vi "Configure.vi"(8 "error in (no error)":errorcluster, 11 "MCCW ACLR in":refnum<class "MCCW ACLR.lvclass">) -> (0 "error out":errorcluster, 3 "MCCW ACLR out":refnum<class "MCCW ACLR.lvclass">)   [LabVIEW 2020, in "MCCW ACLR.lvclass"]
doc: "Configure the measurements paramaters to sweep.\nThis should be a pop up interface invoked by the configure test button on the main panel."
uses:
  MCCW ACLR.lvclass
  MCCW ACLR.lvclass/MCCW ACLR.ctl
  Controls/ACLR configuration.ctl
panel:
  in  "Signal BW [MHz]":dbl
  in  "Number of Carrieres":enum32{"From To", "Array"}(tab)
  in  "Carriers Cluster":cluster{"From":dbl, "To":dbl, "Step":dbl}
  in  "Carriers Array":dbl[](array[numeric]) format="%#_6p"
  in  "OK Button":bool
  in  "Number of Measurements":u32
  in  "MCCW Random Phase":bool
  in  "MCCW Phase Value":dbl min=0.0 max=360.0 step=0.01
  in  "Power":enum32{"From To", "Array"}(tab)
  in  "Power Cluster":cluster{"From":dbl, "To":dbl, "Step":dbl}
  in  "Power Array":dbl[](array[numeric]) format="%#_6p"
  in  "Frequency":enum32{"From To", "Array"}(tab)
  in  "Frequency Cluster":cluster{"From":dbl, "To":dbl, "Step":dbl}
  in  "Frequency Array":dbl[](array[numeric]) format="%#_6p"
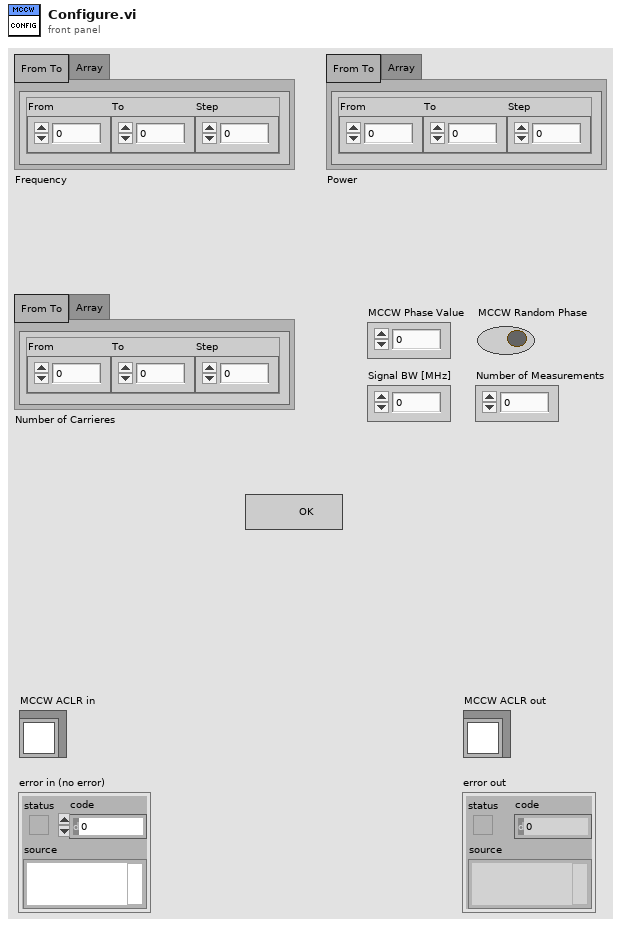
[diagram p1: front panel]
types:
  T1 = enum8{"Enabled", "Disabled", "Disabled and Grayed Out"}
  T2 = typedef "MCCW ACLR.lvclass/ACLR configuration.ctl" = cluster{"Frequency":cluster{"Cluster ":cluster{"From":dbl, "To":dbl, "Step":dbl}, "Array":dbl[], "Use Array":bool}, "Power":cluster{"Cluster ":cluster{"From":dbl, "To":dbl, "Step":dbl}, "Array":dbl[], "Use Array":bool}, "Carriers":cluster{"Cluster ":cluster{"From":dbl, "To":dbl, "Step":dbl}, "Array":dbl[], "Use Array":bool}, "Phase Value":dbl, "Number of Measurements":u32, "Use random phase":bool, "Signal BW [MHz] ":dbl}
  T3 = cluster{"Cluster ":cluster{"From":dbl, "To":dbl, "Step":dbl}, "Array":dbl[], "Use Array":bool}
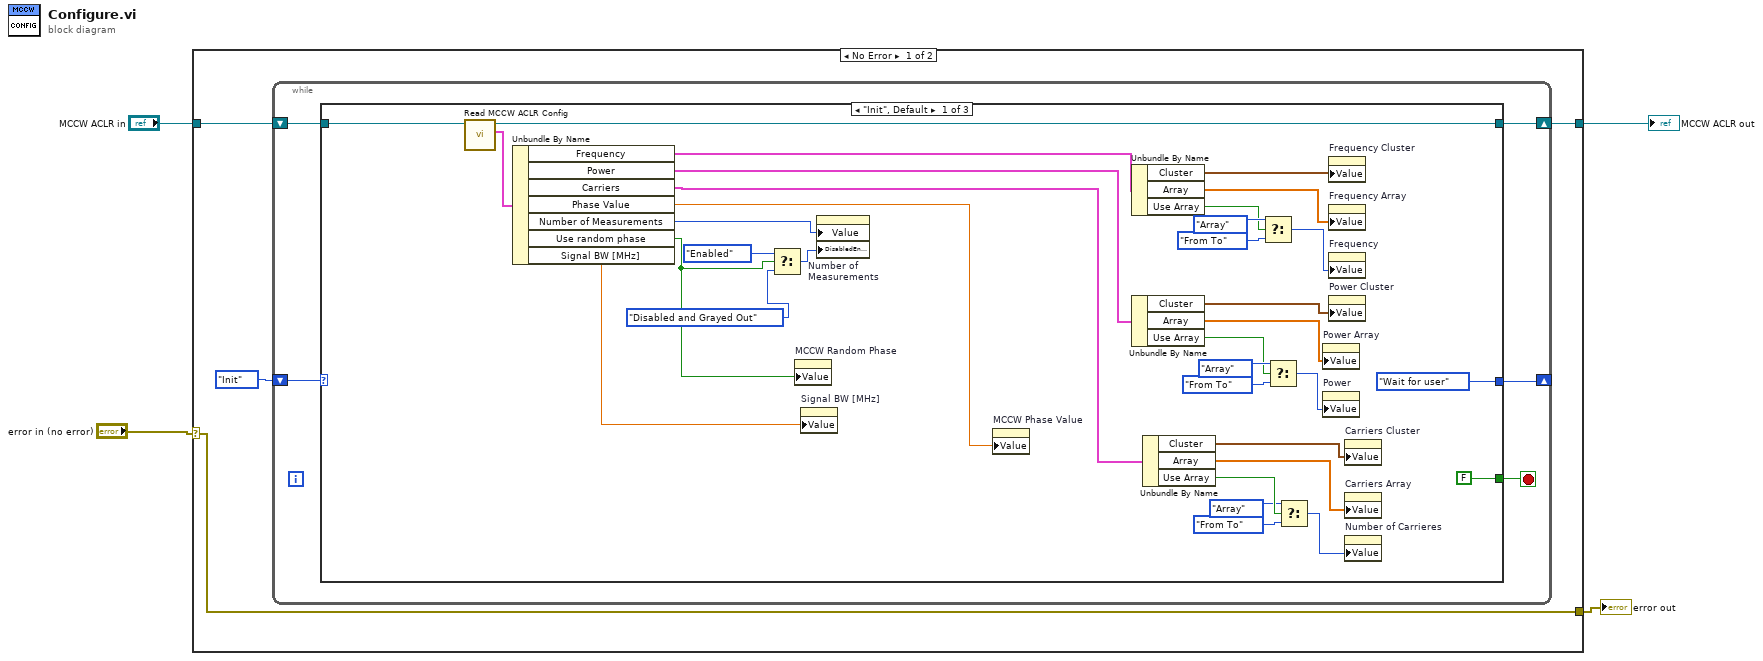
[diagram p0: block diagram]
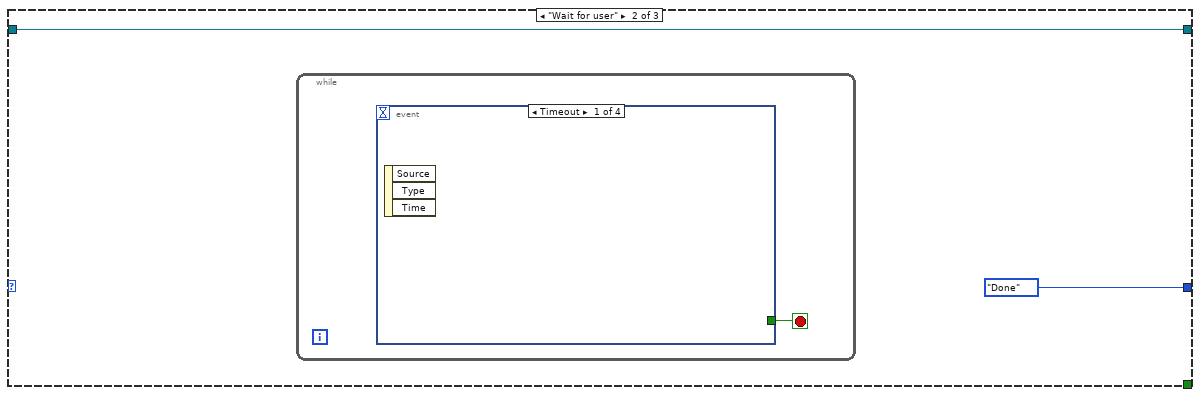
[diagram p2: hidden frame]
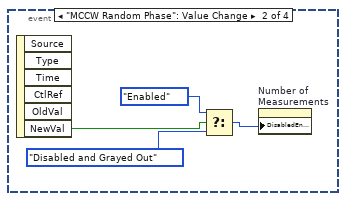
[diagram p3: hidden frame]
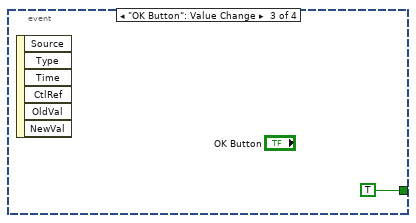
[diagram p4: hidden frame]
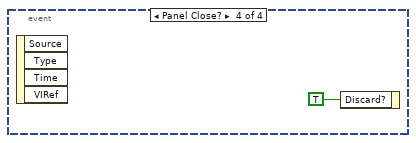
[diagram p5: hidden frame]
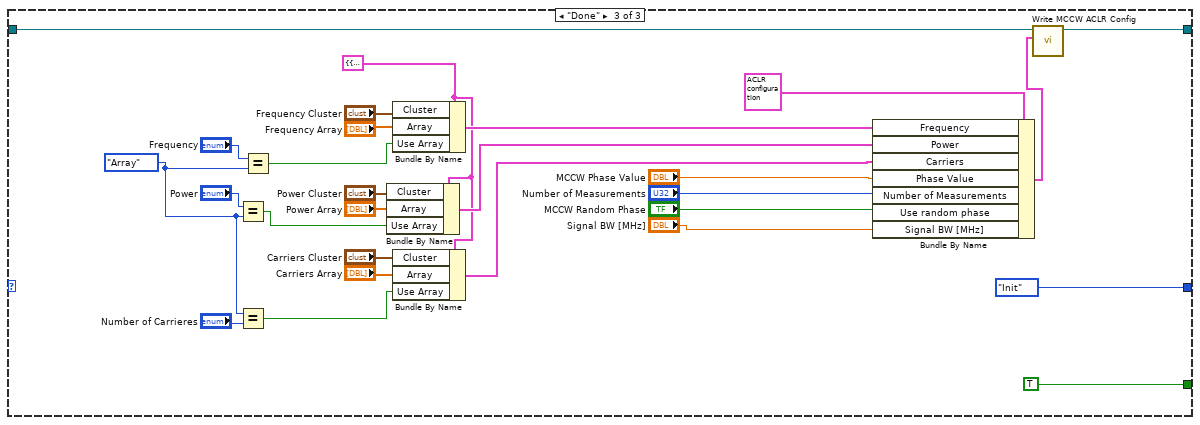
[diagram p6: hidden frame]
diagram:
  n1 = case shown="No Error" "error in (no error)" {
    selector: "error in (no error)" -> [w5 w83]
    tunnel: "MCCW ACLR in" -> [w8 w84]
    tunnel: [w6 w84] -> w2
    tunnel: [w5 w83] -> w1
    frame No Error {
      n2 = while {
        shift-right: [w9] -> w6
        shift-left: w8 -> [w12]
        shift-right: [w11] -> _
        shift-left: enum16{"Init", "Wait for user", "Done"}."Init" -> [w13]
        stop <- w10 stop-if-true
        n3 = case shown="\"Init\", Default" w13 {
          tunnel: w12 -> [w46 w48 w80]
          tunnel: [enum16{"Init", "Wait for user", "Done"}."Wait for user" enum16{"Init", "Wait for user", "Done"}."Done" enum16{"Init", "Wait for user", "Done"}."Init"] -> w11
          tunnel: [FALSE _ TRUE] -> w10
          tunnel: [w22 w48 w79] -> w9
          frame "Init", Default {
            n4 = call "Read MCCW ACLR Config.vi"("MCCW ACLR in"=w46) -> ("MCCW ACLR Config"=w45:T2, "MCCW ACLR out"=w22:refnum<class "MCCW ACLR.lvclass">)  [unwired: 9 in]
            n5 = Unbundle By Name(w45) -> ("Frequency"=w44:T3, "Power"=w41:T3, "Carriers"=w15:T3, "Phase Value"=w30:dbl, "Number of Measurements"=w29:u32, "Use random phase"=w28:bool, "Signal BW [MHz]"=w14:dbl)
            n6 = Select(t=T1."Enabled" ("Disabled"), s=w28, f=T1."Disabled and Grayed Out") -> (s? t:f=w26:T1)
            n7 = property on="MCCW Random Phase" class="Bool (strict)"("Value"=w28) -> ()  [unwired: 2 in, 2 out]
            n8 = property on="Signal BW [MHz]" class="DigNum (strict)"("Value"=w14) -> ()  [unwired: 2 in, 2 out]
            n9 = property on="Number of Measurements" class="DigNum (strict)"("Value"=w29, "DisabledEnum"=w26) -> ()  [unwired: 2 in, 2 out]
            n10 = property on="MCCW Phase Value" class="DigNum (strict)"("Value"=w30) -> ()  [unwired: 2 in, 2 out]
            n11 = Unbundle By Name(w44) -> ("Cluster"=w42:cluster{"From":dbl, "To":dbl, "Step":dbl}, "Array"=w43:dbl[], "Use Array"=w37:bool)
            n12 = Unbundle By Name(w41) -> ("Cluster"=w40:cluster{"From":dbl, "To":dbl, "Step":dbl}, "Array"=w39:dbl[], "Use Array"=w32:bool)
            n13 = Unbundle By Name(w15) -> ("Cluster"=w18:cluster{"From":dbl, "To":dbl, "Step":dbl}, "Array"=w17:dbl[], "Use Array"=w21:bool)
            n14 = Select(t=enum32{"From To", "Array"}."Array" ("Frequency"), s=w37, f=enum32{"From To", "Array"}."From To" ("Frequency")) -> (s? t:f=w35:enum32{"From To", "Array"})
            n15 = Select(t=enum32{"From To", "Array"}."Array" ("Frequency"), s=w32, f=enum32{"From To", "Array"}."From To" ("Frequency")) -> (s? t:f=w31:enum32{"From To", "Array"})
            n16 = Select(t=enum32{"From To", "Array"}."Array" ("Frequency"), s=w21, f=enum32{"From To", "Array"}."From To" ("Frequency")) -> (s? t:f=w16:enum32{"From To", "Array"})
            n17 = property on="Power Array" class="Arr (strict)"("Value"=w39) -> ()  [unwired: 2 in, 2 out]
            n18 = property on="Power" class="TabCtl (strict)"("Value"=w31) -> ()  [unwired: 2 in, 2 out]
            n19 = property on="Frequency Cluster" class="Clust (strict)"("Value"=w42) -> ()  [unwired: 2 in, 2 out]
            n20 = property on="Frequency Array" class="Arr (strict)"("Value"=w43) -> ()  [unwired: 2 in, 2 out]
            n21 = property on="Frequency" class="TabCtl (strict)"("Value"=w35) -> ()  [unwired: 2 in, 2 out]
            n22 = property on="Power Cluster" class="Clust (strict)"("Value"=w40) -> ()  [unwired: 2 in, 2 out]
            n23 = property on="Carriers Cluster" class="Clust (strict)"("Value"=w18) -> ()  [unwired: 2 in, 2 out]
            n24 = property on="Carriers Array" class="Arr (strict)"("Value"=w17) -> ()  [unwired: 2 in, 2 out]
            n25 = property on="Number of Carrieres" class="TabCtl (strict)"("Value"=w16) -> ()  [unwired: 2 in, 2 out]
          }
          frame "Wait for user" {
            n26 = while {
              stop <- w49 stop-if-true
              n27 = event shown="[0] Timeout" {
                selector: _ -> [_ _ _ _]
                dyn-events: _ -> [_ _ _ _]
                timeout: _ -> [_ _ _ _]
                tunnel: [_ _ TRUE _] -> w49
                event Timeout {
                  n28 = event-data() -> ()  [unwired: 1 in, 3 out]
                }
                event "MCCW Random Phase": Value Change {
                  n29 = event-data() -> ("NewVal"=w51:bool)  [unwired: 1 in, 5 out]
                  n30 = Select(t=T1."Enabled" ("Disabled"), s=w51, f=T1."Disabled and Grayed Out") -> (s? t:f=w53:T1)
                  n31 = property on="Number of Measurements" class="DigNum (strict)"("DisabledEnum"=w53) -> ()  [unwired: 2 in, 2 out]
                }
                event "OK Button": Value Change {
                  n32 = event-data() -> ()  [unwired: 1 in, 6 out]
                }
                event Panel Close? {
                  n33 = event-data() -> ()  [unwired: 1 in, 4 out]
                  n34 = event-data("Discard?"=TRUE) -> ()  [unwired: 1 in, 1 out]
                }
              }
            }
          }
          frame "Done" {
            w61 = enum32{"From To", "Array"}."Array" ("y")
            w68 = T3 {"Cluster "={"From"=0.0, "To"=0.0, "Step"=0.0}, "Array"=[], "Use Array"=FALSE} ("Frequency")
            n35 = Equal?(x="Power", y=w61) -> (x = y?=w63:bool)
            n36 = Equal?(x=w61, y="Number of Carrieres") -> (x = y?=w60:bool)
            n37 = Equal?(x="Frequency", y=w61) -> (x = y?=w65:bool)
            n38 = Bundle By Name(cluster=w68, "Cluster"="Power Cluster", "Array"="Power Array", "Use Array"=w63) -> (w74:T3)
            n39 = Bundle By Name(cluster=w68, "Cluster"="Frequency Cluster", "Array"="Frequency Array", "Use Array"=w65) -> (w75:T3)
            n40 = Bundle By Name(cluster=w68, "Cluster"="Carriers Cluster", "Array"="Carriers Array", "Use Array"=w60) -> (w67:T3)
            n41 = Bundle By Name(cluster=T2 {"Frequency"={"Cluster "={"From"=0.0, "To"=0.0, "Step"=0.0}, "Array"=[], "Use Array"=FALSE}, "Power"={"Cluster "={"From"=0.0, "To"=0.0, "Step"=0.0}, "Array"=[], "Use Array"=FALSE}, "Carriers"={"Cluster "={"From"=0.0, "To"=0.0, "Step"=0.0}, "Array"=[], "Use Array"=FALSE}, "Phase Value"=0.0, "Number of Measurements"=0, "Use random phase"=FALSE, "Signal BW [MHz] "=0.0} ("MCCW ACLR Config"), "Frequency"=w75, "Power"=w74, "Carriers"=w67, "Phase Value"="MCCW Phase Value", "Number of Measurements"="Number of Measurements", "Use random phase"="MCCW Random Phase", "Signal BW [MHz]"="Signal BW [MHz]") -> (w59:T2)
            n42 = call "Write MCCW ACLR Config.vi"("MCCW ACLR Config"=w59, "MCCW ACLR in"=w80) -> ("MCCW ACLR out"=w79:refnum<class "MCCW ACLR.lvclass">)  [unwired: 9 in]
          }
        }
      }
    }
    frame Error {
    }
  }
  "error out" <- w1
  "MCCW ACLR out" <- w2
